vi "Queue Ball Element.vi"(11 "Image":T1) -> ()   [LabVIEW 2019]
uses:
  <vilib>/vision/Image Controls.llb/IMAQ Image.ctl
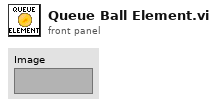
[diagram p1: front panel]
types:
  T1 = typedef "IMAQ Image.ctl" = refnum<image>
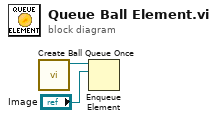
[diagram p0: block diagram]
diagram:
  n1 = call "Create Ball Queue Once.vi"() -> ("queue out"=w1:refnum<queue>)  [unwired: 11 in]
  n2 = Enqueue Element(queue=w1, element="Image") -> ()  [unwired: 2 in, 3 out]
